vi "belt control.vi"(1 "State":T1, 2 "Joystick Z":dbl) -> (0 "output":dbl)   [LabVIEW 2013]
uses:
  typedefs/subStates.ctl
  typedefs/fg_typedef.ctl
panel:
  in  "Time to Wait":u32
  in  "Rate":dbl=0.8 format="%#_13g"
  in  "upper limit":dbl=0.015 format="%#_13g"
  in  "lower limit":dbl=-0.015 format="%#_13g"
  # "Things to Tune"
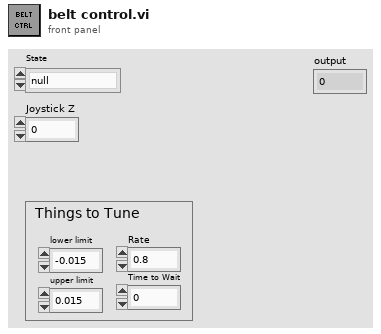
[diagram p1: front panel]
types:
  T1 = typedef "subStates.ctl" = enum16{"null", "wait", "driver control", "auto", "manual override", "hold position", "rotate", "pickup", "pass", "load", "goto shoot", "shoot", "end"}
  T2 = typedef "fg_typedef.ctl" = enum16{"Get", "Set"}
  T3 = typedef "WPI_DigitalInputDevRef.ctl" = cluster{"DevStatus":errorcluster, "DIO Channel":T4, "Digital Module":T5}
  T4 = typedef "FPGA_DIOChannel.ctl" = enum8{"DIO 1", "DIO 2", "DIO 3", "DIO 4", "DIO 5", "DIO 6", "DIO 7", "DIO 8", "DIO 9", "DIO 10", "DIO 11", "DIO 12", "DIO 13", "DIO 14", "Invalid"}
  T5 = typedef "FPGA_TypedefDigitalModule.ctl" = enum16{"Digital Module 1", "Digital Module 2"}
  T6 = typedef "WPI_EncoderDevRef.ctl" = cluster{"DevStatus":errorcluster, "EncoderIndex":T7, "CounterIndex":T8, "DistancePerCount":dbl, "Decoding Type":T9}
  T7 = typedef "FPGA_EncoderIdx.ctl" = enum8{"Enc 0", "Enc 1", "Enc 2", "Enc 3", "Invalid"}
  T8 = typedef "FPGA_CounterCtrSystemIndex.ctl" = enum8{"Ctr 0", "Ctr 1", "Ctr 2", "Ctr 3", "Ctr 4", "Ctr 5", "Ctr 6", "Ctr 7", "Invalid"}
  T9 = typedef "WPI_EncoderType.ctl" = enum16{"1x", "2x", "4x"}
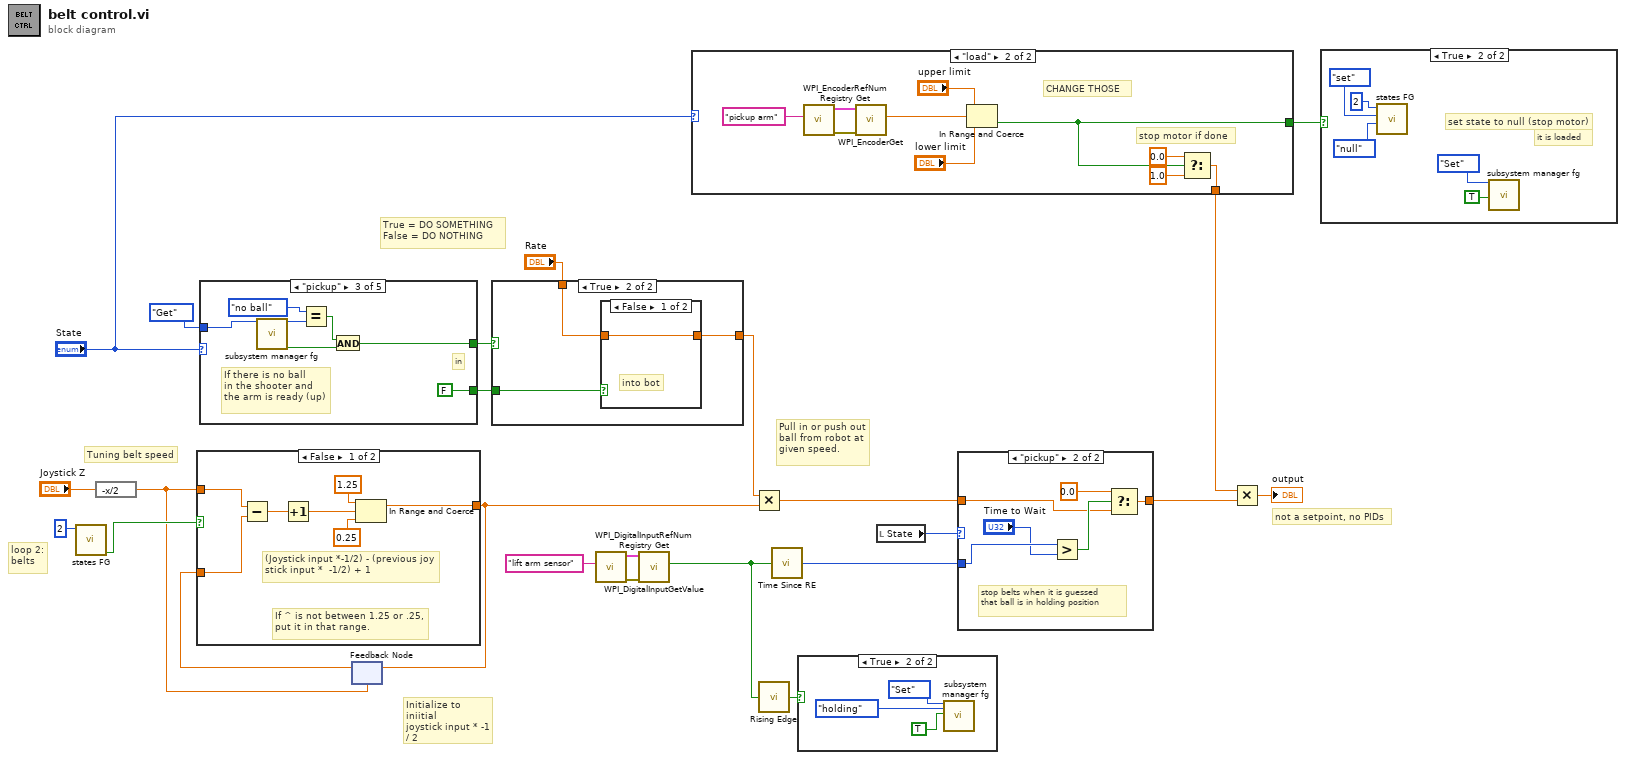
[diagram p0: block diagram]
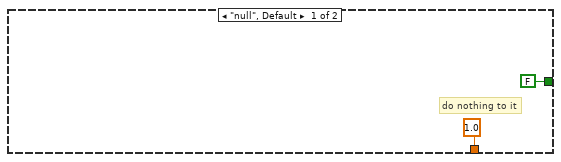
[diagram p4: hidden frame]
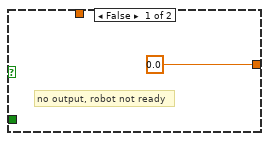
[diagram p6: hidden frame]
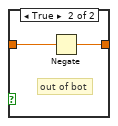
[diagram p7: hidden frame]
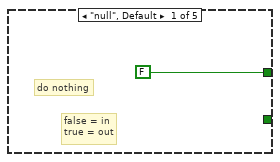
[diagram p8: hidden frame]
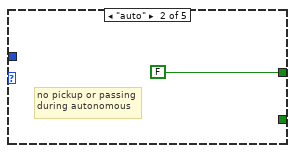
[diagram p9: hidden frame]
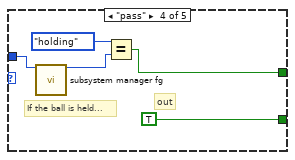
[diagram p10: hidden frame]
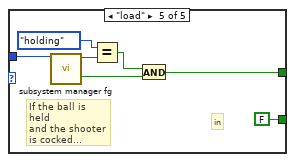
[diagram p11: hidden frame]
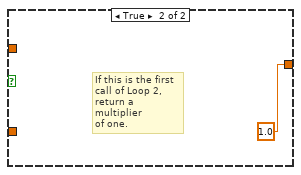
[diagram p12: hidden frame]
diagram:
  # "Pull in or push out\nball from robot at\ngiven speed."
  # "Initialize to iniitial\njoystick input * -1\n/ 2"
  # "True = DO SOMETHING\nFalse = DO NOTHING"
  # "not a setpoint, no PIDs"
  # "Tuning belt speed"
  # "loop 2:\nbelts"
  n1 = call "states FG.vi"("Loop ID"=2) -> ("first call?"=w22:bool)  [unwired: 7 in, 3 out]
  n2 = expression code="-x/2"("Joystick Z") -> (w20:dbl)
  n3 = case shown="\"pickup\"" "State" {
    tunnel: fg_typedef."Get" ("Menu") -> [_ _ w33 w38 w45]
    tunnel: [FALSE ("Arm Ready") FALSE ("Arm Ready") w27 w35 w40] -> w18
    tunnel: [_ _ FALSE TRUE FALSE] -> w15
    frame "null", Default {
      # "false = in\ntrue = out"
      # "do nothing"
    }
    frame "auto" {
      # "no pickup or passing\nduring autonomous"
    }
    frame "pickup" {
      # "in"
      # "If there is no ball\nin the shooter and\nthe arm is ready (up)"
      n4 = call "subsystem manager fg.vi"("Menu"=w33) -> ("Ball State Read"=w30:enum16{"no ball", "holding", "loaded"}, "Arm Ready"=w28:bool)  [unwired: 14 in, 3 out]
      n5 = Equal?(x=enum16{"no ball", "holding", "loaded"}."no ball" ("y"), y=w30) -> (x = y?=w29:bool)
      n6 = And(x=w29, y=w28) -> (x .and. y?=w27:bool)
    }
    frame "pass" {
      # "out"
      # "If the ball is held..."
      n7 = call "subsystem manager fg.vi"("Menu"=w38) -> ("Ball State Read"=w36:enum16{"no ball", "holding", "loaded"})  [unwired: 14 in, 4 out]
      n8 = Equal?(x=enum16{"no ball", "holding", "loaded"}."holding" ("Ball State Read"), y=w36) -> (x = y?=w35:bool)
    }
    frame "load" {
      # "in"
      # "If the ball is held\nand the shooter\nis cocked..."
      n9 = call "subsystem manager fg.vi"("Menu"=w45) -> ("Ball State Read"=w43:enum16{"no ball", "holding", "loaded"}, "Shooter Cocked"=w39:bool)  [unwired: 14 in, 3 out]
      n10 = Equal?(x=enum16{"no ball", "holding", "loaded"}."holding" ("y"), y=w43) -> (x = y?=w41:bool)
      n11 = And(x=w41, y=w39) -> (x .and. y?=w40:bool)
    }
  }
  n12 = feedback #1(w20) -> (w21:dbl)
  n13 = case shown="False" w22 {
    tunnel: [w50 1.0 ("Joystick Z")] -> w16
    tunnel: w21 -> [w46 _]
    tunnel: w20 -> [w47 _]
    frame False {
      # "If ^ is not between 1.25 or .25,\nput it in that range."
      # "(Joystick input *-1/2) - (previous joy\nstick input *  -1/2) + 1"
      n14 = Subtract(x=w47, y=w46) -> (x-y=w48:dbl)
      n15 = Increment(x=w48) -> (x+1=w49:dbl)
      n16 = In Range and Coerce(upper limit=1.25, x=w49, lower limit=0.25) -> (coerced(x)=w50:dbl)  [unwired: 1 out]
    }
    frame True {
      # "If this is the first\ncall of Loop 2,\nreturn a multiplier\nof one."
    }
  }
  n17 = feedback-in #1(w16) -> ()
  n18 = case shown="True" w18 {
    tunnel: [0.0 ("f") w56] -> w17
    tunnel: w15 -> [_ w57]
    tunnel: "Rate" -> [_ w55]
    frame False {
      # "no output, robot not ready"
    }
    frame True {
      n19 = case shown="False" w57 {
        tunnel: [w58 w60] -> w56
        tunnel: w55 -> [w58 w59]
        frame False {
          # "into bot"
        }
        frame True {
          # "out of bot"
          n20 = Negate(x=w59) -> (-x=w60:dbl)
        }
      }
    }
  }
  n21 = call <vilib>:"WPI_DigitalInputRefNum Registry Get.vi"("refnum name"="lift arm sensor") -> ("error out"=w14:errorcluster, "DigitalInputDevRef"=w13:T3)  [unwired: 9 in]
  n22 = call <vilib>:"WPI_DigitalInputGetValue.vi"("error in (no error)"=w14, "DigitalInputDevRef"=w13) -> ("Value"=w7:bool)  [unwired: 7 in, 2 out]
  n23 = case shown="\"load\"" "State" {
    tunnel: [FALSE w65] -> w10
    tunnel: [1.0 w66] -> w8
    frame "null", Default {
      # "do nothing to it"
    }
    frame "load" {
      # "stop motor if done"
      # "CHANGE THOSE"
      n24 = call <vilib>:"WPI_EncoderRefNum Registry Get.vi"("refnum name"="pickup arm") -> ("error out"=w70:errorcluster, "EncoderDevRef"=w71:T6)  [unwired: 9 in]
      n25 = call <vilib>:"WPI_EncoderGet.vi"("error in (no error)"=w70, "EncoderDevRef"=w71) -> ("Distance"=w67:dbl)  [unwired: 4 in, 5 out]
      n26 = In Range and Coerce(upper limit="upper limit", x=w67, lower limit="lower limit") -> (In Range?=w65:bool)  [unwired: 1 out]
      n27 = Select(t=0.0, s=w65, f=1.0) -> (s? t:f=w66:dbl)
    }
  }
  n28 = Multiply(x=w17, y=w16) -> (x*y=w3:dbl)
  n29 = call "Rising Edge.vi"("Input"=w7) -> ("Rising Edge"=w6:bool)
  n30 = call "Time Since RE.vi"("Input"=w7) -> ("Time Since RE of Input"=w1:u32)
  n31 = case shown="True" w6 {
    frame False {
    }
    frame True {
      n32 = call "subsystem manager fg.vi"("Menu"=fg_typedef."Set", "Ball State Write"=enum16{"no ball", "holding", "loaded"}."holding", "Picked Up"=TRUE) -> ()  [unwired: 12 in, 5 out]
    }
  }
  n33 = local read "State"() -> (w4:T1)
  n34 = case shown="\"pickup\"" w4 {
    tunnel: w3 -> [w76 w78]
    tunnel: [w76 w80] -> w2
    tunnel: w1 -> [_ w82]
    frame "null", Default {
    }
    frame "pickup" {
      # "stop belts when it is guessed\nthat ball is in holding position"
      n35 = Greater?(x=w82, y="Time to Wait") -> (0:w79:bool)
      n36 = Select(t=0.0, s=w79, f=w78) -> (s? t:f=w80:dbl)
    }
  }
  n37 = Multiply(x=w8, y=w2) -> (x*y=→"output":dbl)
  n38 = case shown="True" w10 {
    frame False {
    }
    frame True {
      # "it is loaded"
      # "set state to null (stop motor)"
      n39 = call "states FG.vi"("subState in"=subStates."null", "menu (get)"=enum16{"set", "get"}."set", "Loop ID"=2) -> ()  [unwired: 5 in, 4 out]
      n40 = call "subsystem manager fg.vi"("Menu"=fg_typedef."Set", "Loaded"=TRUE) -> ()  [unwired: 13 in, 5 out]
    }
  }
